vi "Read Root Symbol Information.vi"(8 "error in (no error)":errorcluster, 11 "TwinCAT ADS in":refnum<class "TwinCAT ADS.lvclass">) -> (0 "error out":errorcluster, 1 "Symbols Information":T1[](array[typedef]) {"Type ID" items=["ADST_VOID"=0, "ADST_INT16"=2, "ADST_INT32"=3, "ADST_REAL32"=4, "ADST_REAL64"=5, "ADST_INT8"=16, "ADST_UINT8"=17, "ADST_UINT16"=18, "ADST_UINT32"=19, "ADST_INT64"=20, "ADST_UINT64"=21, "ADST_STRING"=30, "ADST_WSTRING"=31, "ADST_REAL80"=32, "ADST_BIT"=33, "ADST_MAXTYPES"=34, "ADST_BIGTYPE"=65]; "Type Category" items=["Unknown, None"=0, "Primitive"=1, "Alias"=2, "Enum"=3, "Array"=4, "Struct"=5, "FunctionBlock"=6, "Program"=7, "Function"=8, "SubRange"=9, "String"=10, "Bitset"=12, "Pointer"=13, "Union"=14, "Reference"=15, "Interface"=16]}, 3 "TwinCAT ADS out":refnum<class "TwinCAT ADS.lvclass">)   [LabVIEW 2018, in "TwinCAT ADS.lvclass"]
uses:
  TwinCAT ADS.lvclass
  Controls/Symbol Information.ctl
  TwinCAT ADS.lvclass/TwinCAT ADS.ctl
  TwinCAT.Ads
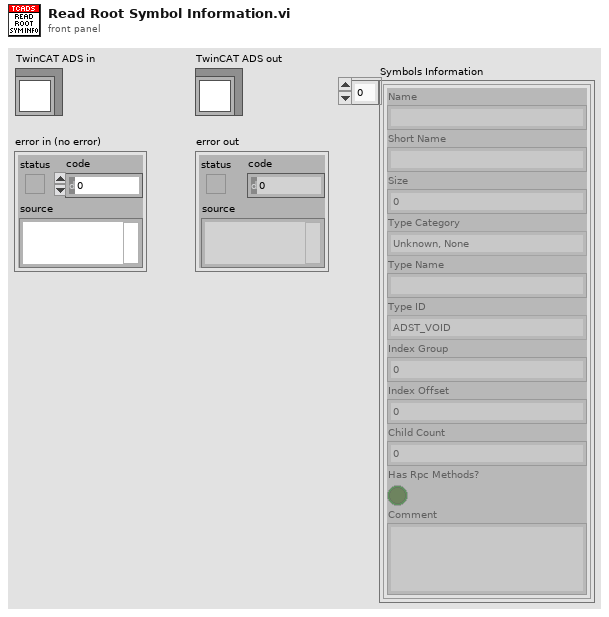
[diagram p1: front panel]
types:
  T1 = typedef "TwinCAT ADS.lvclass/Symbol Information.ctl" = cluster{"Name":string, "Short Name":string, "Size":i32, "Type Category":i32, "Type Name":string, "Type ID":i32, "Index Group":i64, "Index Offset":i64, "Child Count":i32, "Has Rpc Methods?":bool, "Comment":string}
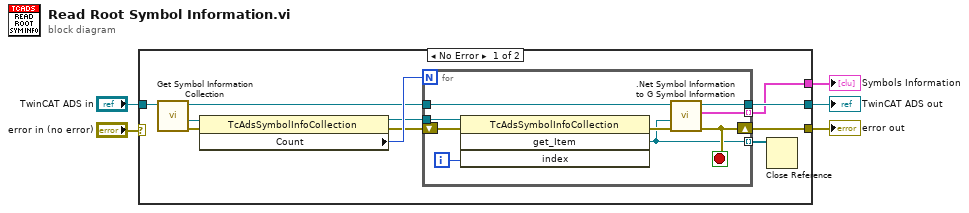
[diagram p0: block diagram]
diagram:
  n1 = case shown="No Error" "error in (no error)" {
    selector: "error in (no error)" -> [_ w27]
    tunnel: [w13 w27] -> w4
    tunnel: [w9 w26] -> w2
    tunnel: "TwinCAT ADS in" -> [w6 w26]
    tunnel: [w8 _] -> w1
    frame No Error {
      n2 = call "Get Symbol Information Collection.vi"("TwinCAT ADS in"=w6) -> ("error out"=w12:errorcluster, ".NET AdsSymbolInfoCollection"=w11:refnum<k24>, "TwinCAT ADS out"=w10:refnum<class "TwinCAT ADS.lvclass">)  [unwired: 8 in]
      n3 = property class="TcAdsSymbolInfoCollection"(reference=w11, error in=w12) -> (reference out=w14:refnum<k24>, error out=w15:errorcluster, "Count"=w16:i32)
      n4 = for {
        N: w16 -> [_]
        tunnel: w14 -> [w25]
        tunnel: [w21] -> w8 mode=indexing
        shift-right: [w20] -> w13
        shift-left: w15 -> [w23]
        tunnel: w10 -> [w19]
        tunnel: [w18] -> w9
        tunnel: [w17] -> w7 mode=indexing
        i -> [w24]
        stop <- w20 stop-if-true
        n5 = invoke class="TcAdsSymbolInfoCollection" method="get_Item"(reference=w25, error in=w23, "index"=w24) -> (error out=w22:errorcluster, "get_Item"=w17:refnum<k24>)  [unwired: 1 in, 2 out]
        n6 = call ".Net Symbol Information to G Symbol Information.vi"("TwinCAT ADS in"=w19, ".NET AdsSymbolInfo"=w17, "error in (no error)"=w22) -> ("TwinCAT ADS out"=w18:refnum<class "TwinCAT ADS.lvclass">, "Symbol Information"=w21:T1, "error out"=w20:errorcluster)  [unwired: 5 in]
      }
      n7 = Close Reference(reference=w7) -> ()  [unwired: 1 in, 1 out]
    }
    frame Error {
    }
  }
  "error out" <- w4
  "TwinCAT ADS out" <- w2
  "Symbols Information" <- w1
